vi "Process.vi"(8 "error in":errorcluster, 11 "Plugin in":refnum<class "Performanced XNET CAN Logger.lvclass">) -> (0 "error out":errorcluster, 3 "Plugin out":refnum<class "Performanced XNET CAN Logger.lvclass">)   [LabVIEW 2021, in "Performanced XNET CAN Logger.lvlib" / "Performanced XNET CAN Logger.lvclass"]
uses:
  Performanced XNET CAN Logger.lvclass
  C:/Program Files/National Instruments/LabVIEW 2021/vi.lib/FlexLogger/SDK/PluginSDK.lvlibp/PEFClasses/SDK/Plugin/Plugin.lvclass
  <vilib>/FlexLogger/SDK/PluginSDK.lvlibp/PEFClasses/SDK/Channel/ParameterAccess/Read Enum.vi
  <vilib>/FlexLogger/SDK/PluginSDK.lvlibp/PEFClasses/SDK/Plugin/DataHelpers/Write 1D DBL (NChan 1Sample).vi
  <vilib>/FlexLogger/SDK/PluginSDK.lvlibp/PEFClasses/SDK/Plugin/Plugin.lvclass
  XNET-CAN-Signal-Logger.lvlib
  <vilib>/FlexLogger/SDK/PluginSDK.lvlibp/PEFClasses/SDK/Channel/Channel.lvclass
  C:/Program Files/National Instruments/LabVIEW 2021/vi.lib/FlexLogger/SDK/PluginSDK.lvlibp/PEFClasses/SDK/Processing Element/Processing Element.lvclass
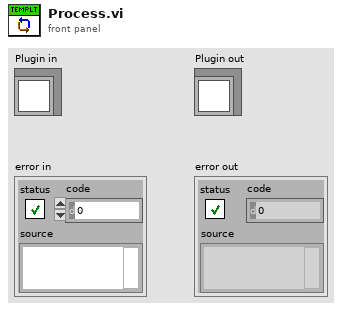
[diagram p1: front panel]
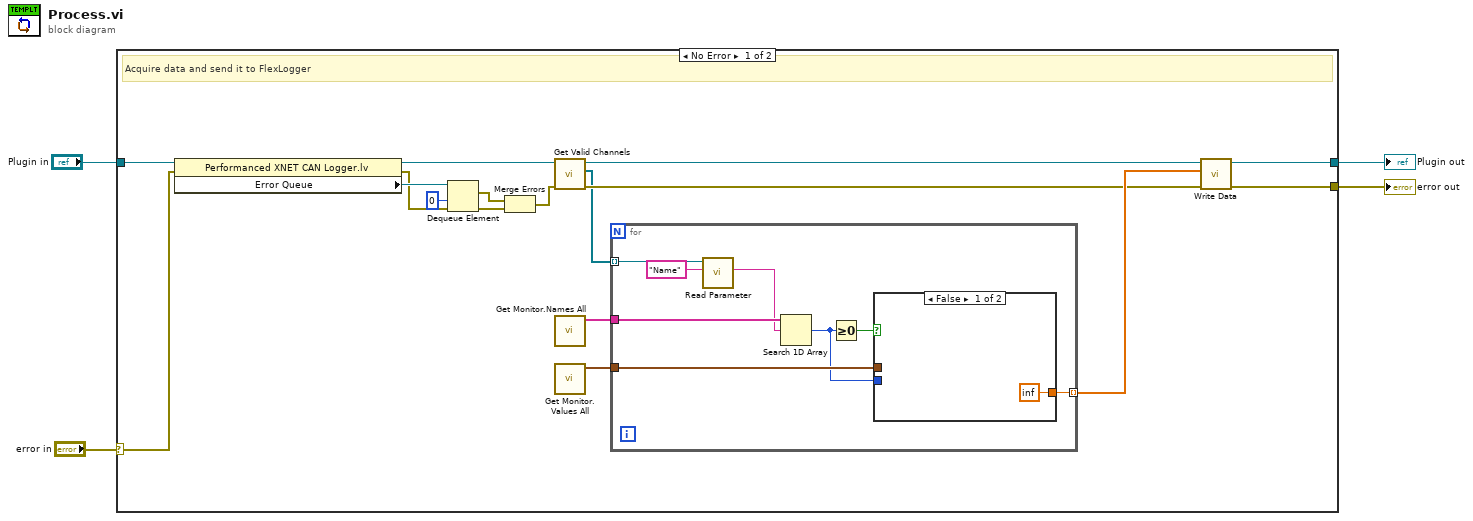
[diagram p0: block diagram]
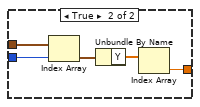
[diagram p2: hidden frame]
diagram:
  n1 = case shown="No Error" "error in" {
    selector: "error in" -> [w17 w36]
    tunnel: [w20 w37] -> w4
    tunnel: "Plugin in" -> [w19 w37]
    tunnel: [w21 w36] -> w1
    frame No Error {
      # "Acquire data and send it to FlexLogger"
      n2 = property class="Performanced XNET CAN Logger.lv"(reference=w19, error in=w17) -> (reference out=w18:refnum<class "Performanced XNET CAN Logger.lvclass">, error out=w15:errorcluster, "Error Queue"=w16:refnum<queue>)
      n3 = Dequeue Element(queue=w16, timeout in ms (-1)=0, error in (no error)=w15) -> (element=w9:errorcluster, error out=w14:errorcluster)  [unwired: 2 out]
      n4 = Merge Errors(w9, w14) -> (w7:errorcluster)
      n5 = call <vilib>:"Get Valid Channels.vi"("error in (no error)"=w7, "Plugin in"=w18) -> ("error out"=w6:errorcluster, "Channels"=w5:refnum<class "Channel.lvclass">[], "Plugin out"=w8:refnum<class "Performanced XNET CAN Logger.lvclass">)  [unwired: 7 in]
      n6 = call "Get Monitor.Names All.vi"() -> ("Signal Names"=w12:string[])  [unwired: 10 in, 1 out]
      n7 = call "Get Monitor.Values All.vi"() -> ("Signal Data"=w11:waveform(dbl)[])  [unwired: 10 in, 1 out]
      n8 = for {
        tunnel: w12 -> [w29]
        tunnel: w11 -> [w28]
        tunnel: [w27] -> w10 mode=indexing
        tunnel: w5 -> [w26] mode=indexing
        n9 = call-poly <vilib>:"Read Parameter.vi"("Name"="Name", "Channel in"=w26) -> ("Value"=w24:string)  [unwired: 5 in, 4 out]
        n10 = Search 1D Array(1D array=w29, element=w24) -> (index of element=w22:i32)  [unwired: 1 in]
        n11 = Greater Or Equal To 0?(x=w22) -> (x >= 0?=w23:bool)
        n12 = case shown="False" w23 {
          tunnel: w28 -> [_ w35]
          tunnel: w22 -> [_ w34]
          tunnel: [inf w31] -> w27
          frame False {
          }
          frame True {
            n13 = Index Array(array=w35, index=w34) -> (element=w33:waveform(dbl))
            n14 = Unbundle By Name(w33) -> ("Y"=w32:dbl[])
            n15 = Index Array(array=w32) -> (element=w31:dbl)  [unwired: 1 in]
          }
        }
      }
      n16 = call-poly <vilib>:"Write Data.vi"("error in (no error)"=w6, "Data"=w10, "Plugin in"=w8) -> ("error out"=w21:errorcluster, "Plugin out"=w20:refnum<class "Performanced XNET CAN Logger.lvclass">)  [unwired: 7 in]
    }
    frame Error {
    }
  }
  "error out" <- w1
  "Plugin out" <- w4
